vi "auto extend test.vi"() -> ()   [LabVIEW 2015]
uses:
  <vilib>/Rock Robotics/WPI/MotorControl/WPI_MotorControlDeviceRef.ctl
  <vilib>/Rock Robotics/WPI/MotorControl/WPI_MotorControlType.ctl
  <vilib>/Rock Robotics/SystemInterfaces/DIO/FPGA_DIOPWMChannel.ctl
  <vilib>/Rock Robotics/WPI/PWM/WPI_PWMDeadband.ctl
  <vilib>/Rock Robotics/WPI/CAN/Jaguar/SubVIs/WPI_CANJaguar_ControlMode.ctl
  <vilib>/Rock Robotics/WPI/CAN/TalonSRX/WPI_CANTalonSRX_APIControlMode.ctl
panel:
  out "Scissor Motor Set":dbl
  out "Hook Motor set":dbl
  in  "Hook Encoder Rate":dbl
  in  "Hook Motor":T1={"DeviceStatus"={"status"=FALSE, "code"=0, "source"=""}, "Type"=enum."PWM", "PWM"={"PWM Channel"=enum."Invalid", "DeadBand"={"Name"="", "maxPositivePwm"=0, "minPositivePwm"=0, "centerPwm"=0, "maxNegativePwm"=0, "minNegativePwm"=0, "angularRange"=0}}, "CAN"={"Device Number"=0, "Control Mode"=enum."Percent VBus", "Semaphore"=refnum, "Max Vout"=12.0, "TalonSRX Control Mode"=enum."Percent VBus"}, "Invert"=FALSE}
  in  "Scissor Motor":T1={"DeviceStatus"={"status"=FALSE, "code"=0, "source"=""}, "Type"=enum."PWM", "PWM"={"PWM Channel"=enum."Invalid", "DeadBand"={"Name"="", "maxPositivePwm"=0, "minPositivePwm"=0, "centerPwm"=0, "maxNegativePwm"=0, "minNegativePwm"=0, "angularRange"=0}}, "CAN"={"Device Number"=0, "Control Mode"=enum."Percent VBus", "Semaphore"=refnum, "Max Vout"=12.0, "TalonSRX Control Mode"=enum."Percent VBus"}, "Invert"=FALSE}
  in  "Scissor Encoder Dist":dbl
  in  "Boolean":bool
  out "Cases":T8(ring)
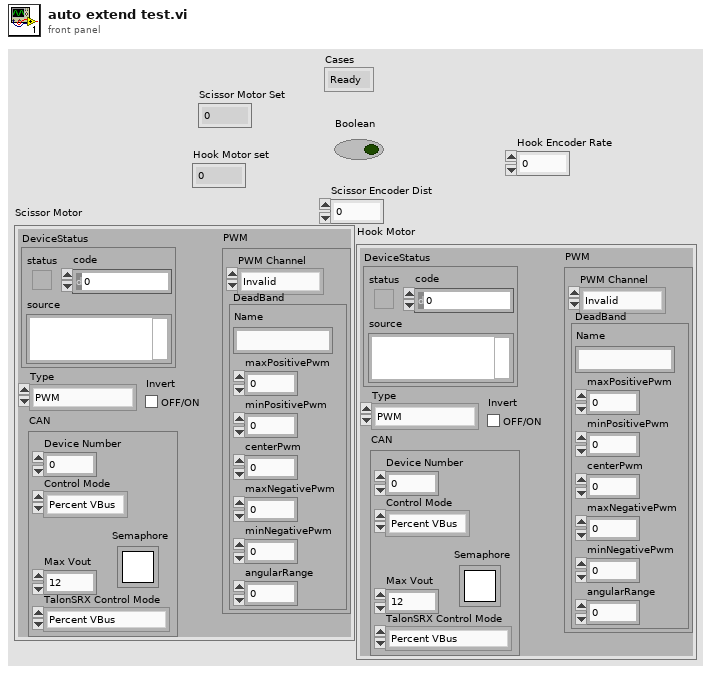
[diagram p1: front panel]
types:
  T1 = typedef "WPI_MotorControlDeviceRef.ctl" = cluster{"DeviceStatus":errorcluster, "Type":T2, "PWM":cluster{"PWM Channel":T3, "DeadBand":T4}, "CAN":cluster{"Device Number":u8, "Control Mode":T5, "Semaphore":T6, "Max Vout":dbl, "TalonSRX Control Mode":T7}, "Invert":bool}
  T2 = typedef "WPI_MotorControlType.ctl" = enum16{"PWM", "CAN", "CANTalonSRX"}
  T3 = typedef "FPGA_DIOPWMChannel.ctl" = enum8{"PWM 0", "PWM 1", "PWM 2", "PWM 3", "PWM 4", "PWM 5", "PWM 6", "PWM 7", "PWM 8", "PWM 9", "PWM MXP 0", "PWM MXP 1", "PWM MXP 2", "PWM MXP 3", "PWM MXP 4", "PWM MXP 5", "PWM MXP 6", "PWM MXP 7", "PWM MXP 8", "PWM MXP 9", "Invalid"}
  T4 = typedef "WPI_PWMDeadband.ctl" = cluster{"Name":string, "maxPositivePwm":i32, "minPositivePwm":i32, "centerPwm":i32, "maxNegativePwm":i32, "minNegativePwm":i32, "angularRange":u16}
  T5 = typedef "WPI_CANJaguar_ControlMode.ctl" = enum8{"Percent VBus", "Current", "Speed", "Position", "Voltage"}
  T6 = typedef "Semaphore RefNum" = refnum<k1>
  T7 = typedef "WPI_CANTalonSRX_APIControlMode.ctl" = enum8{"Percent VBus", "Speed", "Position", "Slave", "Unchanged / Invalid", "Voltage Compensation", "Current", "Motion Profile"}
  T8 = enum16{"Ready", "Extend Lift", "Extend Hook", "Retract Lift", "Hold"}
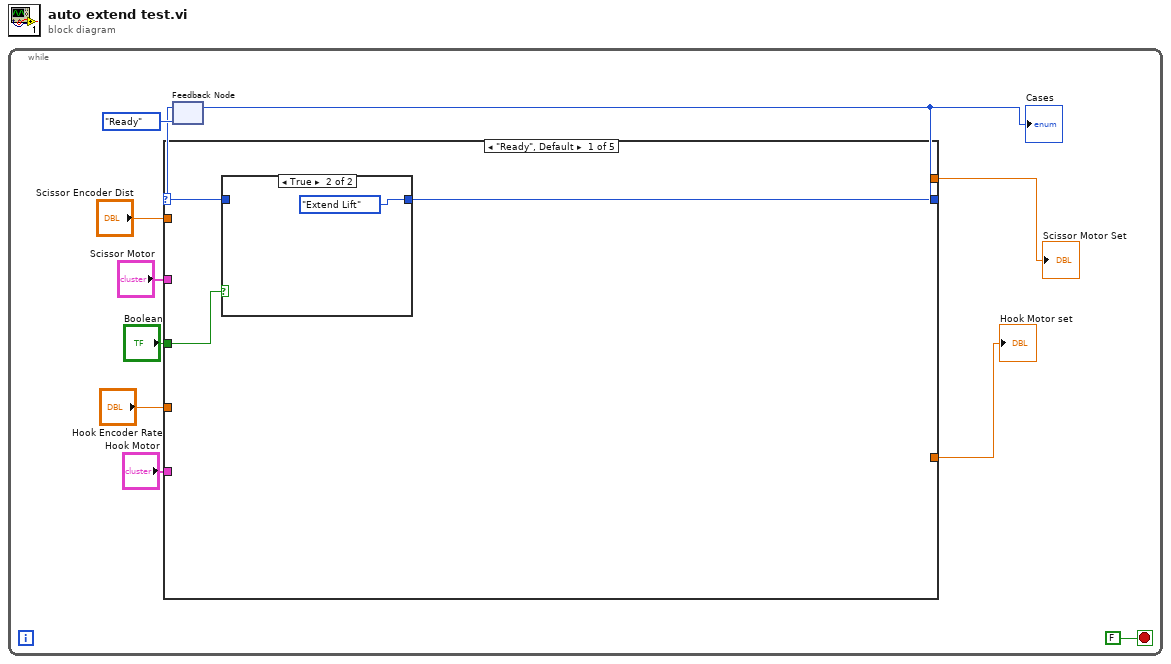
[diagram p0: block diagram]
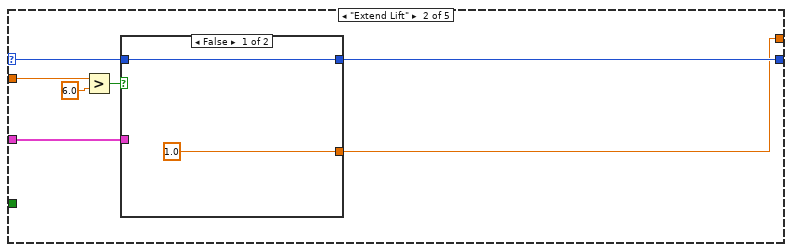
[diagram p3: hidden frame]
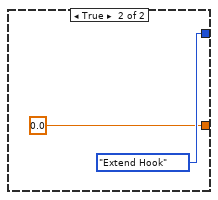
[diagram p4: hidden frame]
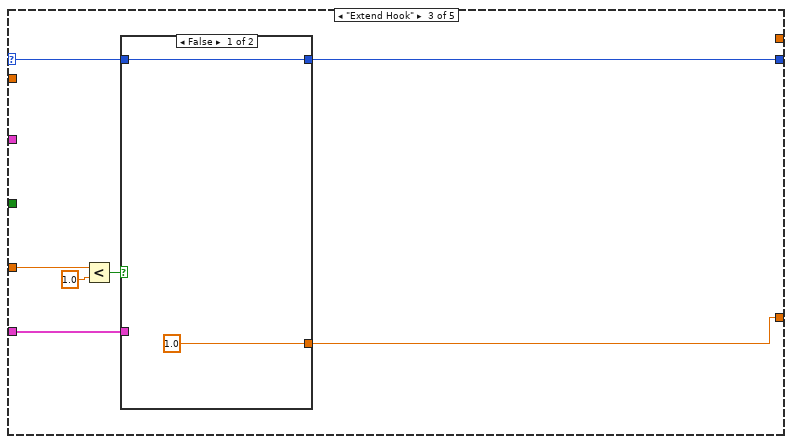
[diagram p5: hidden frame]
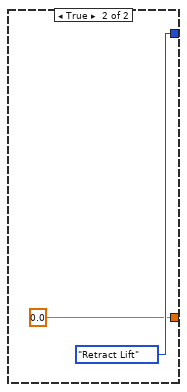
[diagram p6: hidden frame]
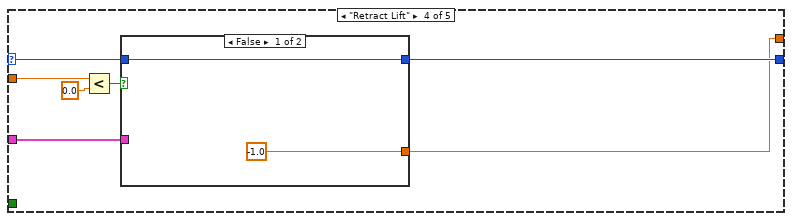
[diagram p7: hidden frame]
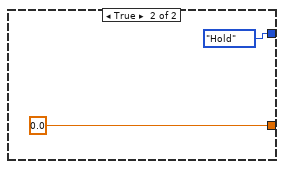
[diagram p8: hidden frame]
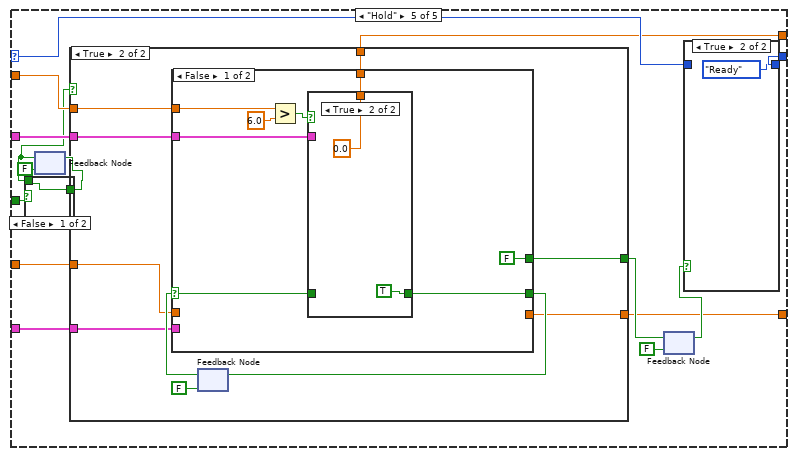
[diagram p9: hidden frame]
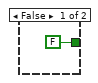
[diagram p11: hidden frame]
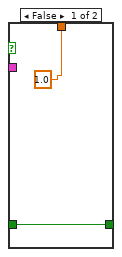
[diagram p12: hidden frame]
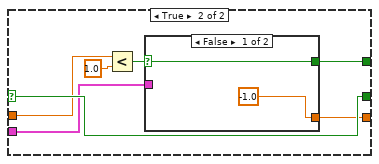
[diagram p13: hidden frame]
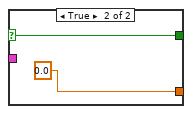
[diagram p14: hidden frame]
diagram:
  n1 = while {
    stop <- FALSE stop-if-true
    n2 = feedback #1(T8."Ready" ("Cases")) -> (w10:T8)
    n3 = case shown="\"Ready\", Default" w10 {
      selector: w10 -> [w14 w22 w34 w45 w64]
      tunnel: [w13 w23 w33 w44 w63] -> w1
      tunnel: "Boolean" -> [w12 _ _ _ w55]
      tunnel: "Scissor Encoder Dist" -> [_ w21 _ w42 w61]
      tunnel: "Scissor Motor" -> [_ w18 _ w43 w60]
      tunnel: "Hook Encoder Rate" -> [_ _ w31 _ w62]
      tunnel: "Hook Motor" -> [_ _ w29 _ w59]
      tunnel: [_ _ w28 _ w51] -> w4
      tunnel: [_ w17 _ w39 w50] -> w3
      frame "Ready", Default {
        n4 = case shown="True" w12 {
          tunnel: [w15 T8."Extend Lift" ("Cases")] -> w13
          tunnel: w14 -> [w15 _]
          frame False {
          }
          frame True {
          }
        }
      }
      frame "Extend Lift" {
        n5 = Greater?(x=w21, y=6.0) -> (0:w19:bool)
        n6 = case shown="False" w19 {
          tunnel: [w25 T8."Extend Hook" ("Cases")] -> w23
          tunnel: w22 -> [w25 _]
          tunnel: w18 -> [_ _]
          tunnel: [1.0 ("Output") 0.0 ("Output")] -> w17
          frame False {
          }
          frame True {
          }
        }
      }
      frame "Extend Hook" {
        n7 = Less?(x=w31, y=1.0) -> (x < y?=w30:bool)
        n8 = case shown="False" w30 {
          tunnel: [w36 T8."Retract Lift" ("Cases")] -> w33
          tunnel: w34 -> [w36 _]
          tunnel: w29 -> [_ _]
          tunnel: [1.0 ("Output") 0.0 ("Output")] -> w28
          frame False {
          }
          frame True {
          }
        }
      }
      frame "Retract Lift" {
        n9 = Less?(x=w42, y=0.0) -> (x < y?=w40:bool)
        n10 = case shown="False" w40 {
          tunnel: [w47 T8."Hold" ("Cases")] -> w44
          tunnel: w45 -> [w47 _]
          tunnel: w43 -> [_ _]
          tunnel: [-1.0 ("Output") 0.0 ("Output")] -> w39
          frame False {
          }
          frame True {
          }
        }
      }
      frame "Hold" {
        n11 = feedback #2(FALSE) -> (w52:bool)
        n12 = case shown="False" w55 {
          selector: w55 -> [_ w66]
          tunnel: [w65 w66] -> w54
          tunnel: w52 -> [w65 _]
          frame False {
          }
          frame True {
          }
        }
        n13 = feedback-in #2(w54) -> ()
        n14 = case shown="True" w52 {
          tunnel: w62 -> [_ w72]
          tunnel: w61 -> [_ w74]
          tunnel: w60 -> [_ w73]
          tunnel: w59 -> [_ w71]
          tunnel: [FALSE w70] -> w58
          tunnel: [_ w69] -> w51
          tunnel: [_ w68] -> w50
          frame False {
          }
          frame True {
            n15 = feedback #3(FALSE) -> (w77:bool)
            n16 = case shown="False" w77 {
              selector: w77 -> [w84 w96]
              tunnel: [w85 w96] -> w75
              tunnel: w74 -> [w83 _]
              tunnel: w73 -> [w80 _]
              tunnel: w72 -> [_ w95]
              tunnel: w71 -> [_ w93]
              tunnel: [FALSE w91] -> w70
              tunnel: [_ w90] -> w69
              tunnel: [w78 _] -> w68
              frame False {
                n17 = Greater?(x=w83, y=6.0) -> (0:w81:bool)
                n18 = case shown="True" w81 {
                  tunnel: [w87 TRUE] -> w85
                  tunnel: w84 -> [w87 _]
                  tunnel: w80 -> [_ _]
                  tunnel: [1.0 ("Output") 0.0 ("Output")] -> w78
                  frame False {
                  }
                  frame True {
                  }
                }
              }
              frame True {
                n19 = Less?(x=w95, y=1.0) -> (x < y?=w92:bool)
                n20 = case shown="False" w92 {
                  selector: w92 -> [w98 w100]
                  tunnel: w93 -> [_ _]
                  tunnel: [w98 w100] -> w91
                  tunnel: [-1.0 ("Output") 0.0 ("Output")] -> w90
                  frame False {
                  }
                  frame True {
                  }
                }
              }
            }
            n21 = feedback-in #3(w75) -> ()
          }
        }
        n22 = feedback-in #4(w58) -> ()
        n23 = feedback #4(FALSE) -> (w57:bool)
        n24 = case shown="True" w57 {
          tunnel: [w101 T8."Ready" ("Cases")] -> w63
          tunnel: w64 -> [w101 _]
          frame False {
          }
          frame True {
          }
        }
      }
    }
    "Cases" <- w1
    "Hook Motor set" <- w4
    "Scissor Motor Set" <- w3
    n25 = feedback-in #1(w1) -> ()
  }
